vi "TPNT_GetValues.vi"(9 "UTC":bool, 10 "device":string="ALL", 11 "Objects":T1[](array[typedef])) -> (1 "names":string, 2 "full out":string)   [LabVIEW 2016]
uses:
  TPNT_Refnum.ctl
  TPNT_CoreFunction.ctl
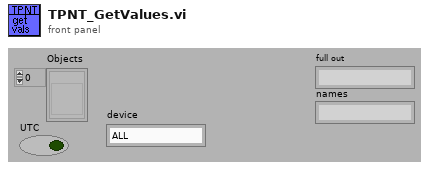
[diagram p1: front panel]
types:
  T1 = typedef "TPNT_Refnum.ctl" = refnum<vi>
  T2 = typedef "TPNT_CoreFunction.ctl" = enum16{"Reset", "Register", "Get Data", "Set Data", "Unregister", "Test", "Get Objects"}
  T3 = typedef "TPNT_DeviceTPs.ctl" = cluster{"device":string, "devupdate":dbl, "next_update":u32, "devinterface":string, "TPs":T4[], "Alarms":bool, "monitor":bool, "log sep":string}
  T4 = typedef "TPNT_TP.ctl" = cluster{"name":string, "type":string, "algor":string[], "update_rate":sgl, "Limits":T5, "Samples":T6, "next_update":u32, "Status":string, "monitor":bool, "error":bool, "Log":T7, "permissions":string, "ID":string}
  T5 = typedef "TPNT_Limits.ctl" = cluster{"Alarm Type":string, "Lower ":dbl, "Upper":dbl, "Nominal":dbl, "outrange":bool, "Check":bool, "latch":bool, "level":string}
  T6 = typedef "TPNT_Samples.ctl" = cluster{"samples":i32, "counter":i32, "Values":dbl[], "Current Value":string, "filter":string, "precision":u8}
  T7 = typedef "TPNT_Log.ctl" = cluster{"log":bool, "file":path, "type":string, "format":string, "updaterate":dbl, "nex_update":u32, "mode":string}
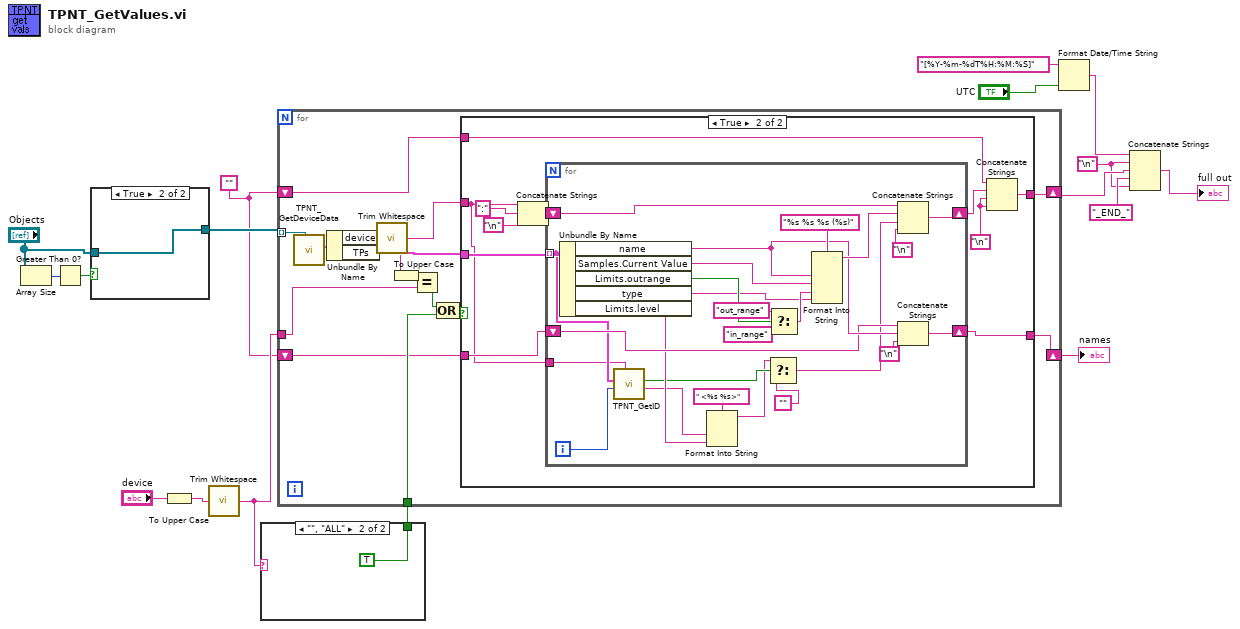
[diagram p0: block diagram]
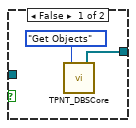
[diagram p2: hidden frame]
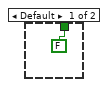
[diagram p3: hidden frame]
diagram:
  w7 = "\n"
  w3 = ""
  n1 = Array Size(array="Objects") -> (size(s)=w6:i32)
  n2 = Greater Than 0?(x=w6) -> (x > 0?=w5:bool)
  n3 = case shown="True" w5 {
    tunnel: [w18 w20] -> w17
    tunnel: "Objects" -> [_ w20]
    frame False {
      n4 = call "TPNT_DBSCore.vi"("Function (Get Data)"=TPNT_CoreFunction."Get Objects") -> ("Objects"=w18:T1[])  [unwired: 4 in, 14 out]
    }
    frame True {
    }
  }
  n5 = To Upper Case(1:"device") -> (0:w10:string)
  n6 = call <vilib>:"Trim Whitespace.vi"("string"=w10) -> ("trimmed string"=w12:string)  [unwired: 1 in]
  n7 = case shown="\"\", \"ALL\"" w12 {
    tunnel: [FALSE TRUE] -> w11
    frame Default {
    }
    frame "", "ALL" {
    }
  }
  n8 = for {
    tunnel: w17 -> [w36] mode=indexing
    shift-right: [w33] -> w8
    shift-left: w3 -> [w32]
    tunnel: w12 -> [w30]
    tunnel: w11 -> [w27]
    shift-right: [w24] -> w2
    shift-left: w3 -> [w23]
    n9 = call "TPNT_GetDeviceData.vi"("Object Refnum In"=w36) -> ("Object Data Out"=w35:T3)  [unwired: 1 in, 9 out]
    n10 = Unbundle By Name(w35) -> ("device"=w31:string, "TPs"=w34:T4[])
    n11 = call <vilib>:"Trim Whitespace.vi"("string"=w31) -> ("trimmed string"=w25:string)  [unwired: 1 in]
    n12 = To Upper Case(1:w25) -> (0:w26:string)
    n13 = Equal?(x=w26, y=w30) -> (x = y?=w29:bool)
    n14 = Compound Arithmetic op=OR(w29, w27) -> (w28:bool)
    n15 = case shown="True" w28 {
      tunnel: w34 -> [_ w49]
      tunnel: [w38 w44] -> w33
      tunnel: w32 -> [w38 w43]
      tunnel: w25 -> [_ w39]
      tunnel: [w37 w41] -> w24
      tunnel: w23 -> [w37 w40]
      frame False {
      }
      frame True {
        w42 = "\n"
        n16 = Concatenate Strings(w39, ":" ("string"), "\n") -> (w48:string)
        n17 = for {
          tunnel: w49 -> [w56] mode=indexing
          shift-right: [w70] -> w45
          shift-left: w48 -> [w71]
          shift-right: [w66] -> w41
          shift-left: w40 -> [w64]
          tunnel: w39 -> [w50]
          i -> [w51]
          n18 = Unbundle By Name(w56) -> ("name"=w65:string, "Samples.Current Value"=w74:string, "Limits.outrange"=w69:bool, "type"=w63:string, "Limits.level"=w59:string)
          n19 = call "TPNT_GetID.vi"("device"=w50, "index in"=w51, "testpoint In"=w56) -> ("id out"=w54:string, "id?"=w55:bool)  [unwired: 7 out]
          n20 = Format Into String(format string=" <%s %s>", w54, w59) -> (resulting string=w53:string)  [unwired: 2 in, 1 out]
          n21 = Select(t=w53, s=w55, f="") -> (s? t:f=w57:string)
          n22 = Select(t="out_range", s=w69, f="in_range") -> (s? t:f=w67:string)
          n23 = Format Into String(format string="%s %s %s (%s)", w65, w74, w67, w63) -> (resulting string=w72:string)  [unwired: 2 in, 1 out]
          n24 = Concatenate Strings(w71, w72, w57, "\n") -> (w70:string)
          n25 = Concatenate Strings(w64, w65, "\n") -> (w66:string)
        }
        n26 = Concatenate Strings(w43, w45, w42, w42) -> (w44:string)
      }
    }
  }
  "names" <- w2
  n27 = Format Date/Time String(time format string (%c)="[%Y-%m-%dT%H:%M:%S]", UTC format="UTC") -> (date/time string=w15:string)  [unwired: 1 out]
  n28 = Concatenate Strings(w15, w7, w8, "_END_" ("string"), w7) -> (→"full out":string)
